vi "auto info.vi"(1 "Autonomous Mode":T1(radio)=enum."Autonomous 1 (Drive)") -> (0 "About Selected Auto Mode":string)   [LabVIEW 2015]
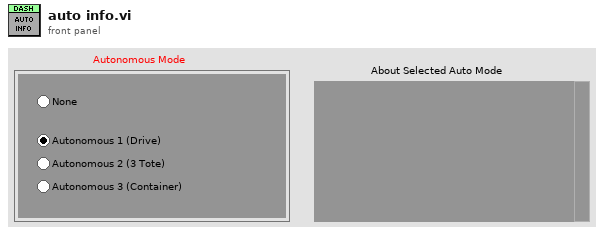
[diagram p1: front panel]
types:
  T1 = enum32{"None", "Autonomous 1 (Drive)", "Autonomous 2 (3 Tote)", "Autonomous 3 (Container)"}
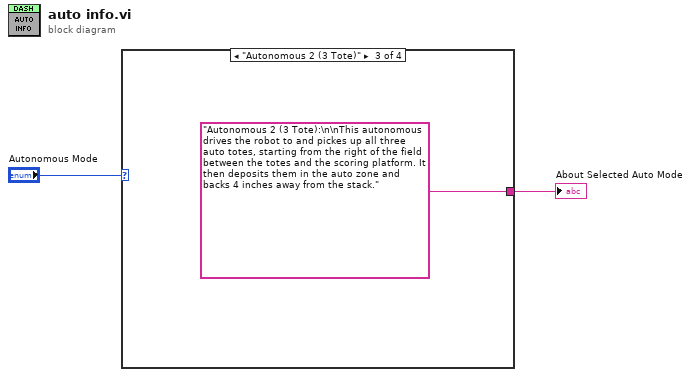
[diagram p0: block diagram]
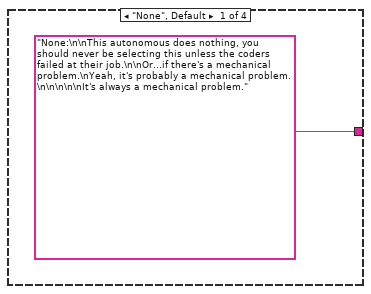
[diagram p2: hidden frame]
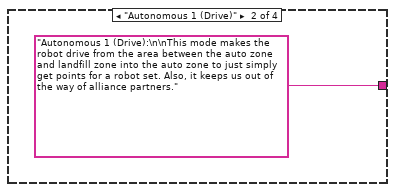
[diagram p3: hidden frame]
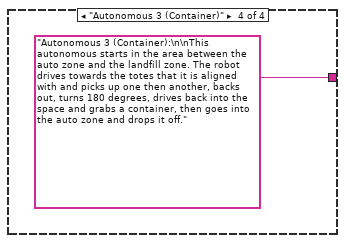
[diagram p4: hidden frame]
diagram:
  n1 = case shown="\"Autonomous 2 (3 Tote)\"" "Autonomous Mode" {
    tunnel: ["None:\n\nThis autonomous does nothing, you should never be selecting this unless the coders failed at their job.\n\nOr...if there's a mechanical problem.\nYeah, it's probably a mechanical problem.\n\n\n\n\nIt's always a mechanical problem." "Autonomous 1 (Drive):\n\nThis mode makes the robot drive from the area between the auto zone and landfill zone into the auto zone to just simply get points for a robot set. Also, it keeps us out of the way of alliance partners." "Autonomous 2 (3 Tote):\n\nThis autonomous drives the robot to and pickes up all three auto totes, starting from the right of the field between the totes and the scoring platform. It then deposits them in the auto zone and backs 4 inches away from the stack." "Autonomous 3 (Container):\n\nThis autonomous starts in the area between the auto zone and the landfill zone. The robot drives towards the totes that it is aligned with and picks up one then another, backs out, turns 180 degrees, drives back into the space and grabs a container, then goes into the auto zone and drops it off."] -> w1
    frame "None", Default {
    }
    frame "Autonomous 1 (Drive)" {
    }
    frame "Autonomous 2 (3 Tote)" {
    }
    frame "Autonomous 3 (Container)" {
    }
  }
  "About Selected Auto Mode" <- w1
